vi "_initialize_amp_phas.vi"(11 "Measurement Frequencies":dbl[](array[numeric])) -> (3 "Initialized Amp/Phas":dbl[][](array[numeric]))   [LabVIEW 2020, in "Resonance Curve Data.lvclass"]
uses:
  Resonance Curve Data.lvclass
panel:
  # "Given 1D array of measurement frequencies, create a corresponding 2D array to store amplitude and phases.\nThe ampliture/phase array is initialized to NaN."
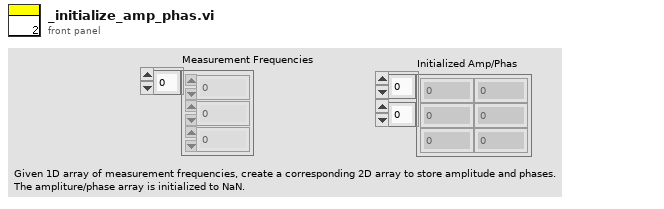
[diagram p1: front panel]
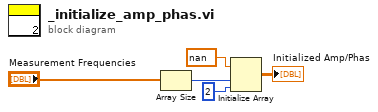
[diagram p0: block diagram]
diagram:
  n1 = Array Size(array="Measurement Frequencies") -> (size(s)=w3:i32)
  n2 = Initialize Array(nan, w3, 2) -> (→"Initialized Amp/Phas":dbl[][])
